vi "test Shutter.vi"() -> ()   [LabVIEW 2014]
doc: "Newport Motion Controler\nThis program test Shutter operations\n\nAndré Romero - 2020\nandretec@ifsc.usp.br"
panel:
  in  "Stop Button":bool
  in  "toggle Shutter":bool
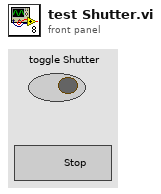
[diagram p1: front panel]
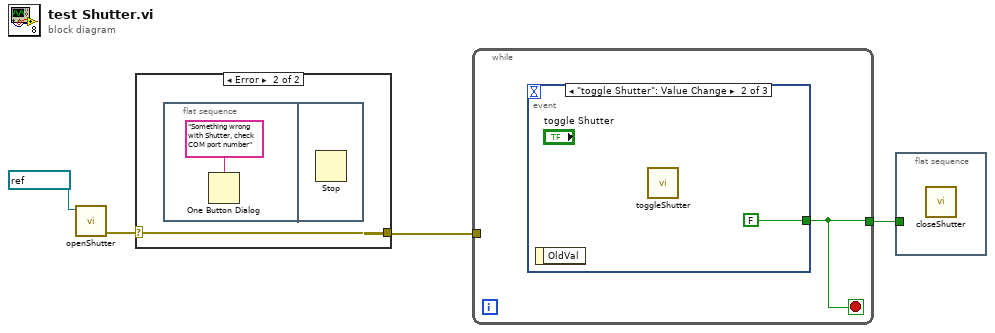
[diagram p0: block diagram]
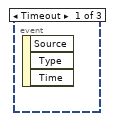
[diagram p2: hidden frame]
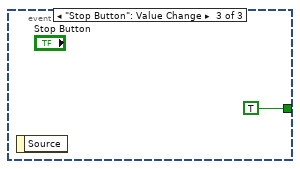
[diagram p3: hidden frame]
diagram:
  n1 = call "openShutter.vi"("VISA Refnum in"=refnum<visa-resource-name> "COM3") -> ("error out"=w3:errorcluster)  [unwired: 9 in, 1 out]
  n2 = case shown="Error" w3 {
    selector: w3 -> [w5 w6]
    tunnel: [w5 w6] -> w2
    frame No Error {
    }
    frame Error {
      n3 = flat-sequence {
        frame #0 {
          n4 = One Button Dialog(message="Something wrong with Shutter, check COM port number") -> ()  [unwired: 1 in, 1 out]
        }
        frame #1 {
          n5 = Stop() -> ()  [unwired: 1 in]
        }
      }
    }
  }
  n6 = while {
    tunnel: w2 -> [_]
    tunnel: [w8] -> w1
    stop <- w8 stop-if-true
    n7 = event shown="[1] \"toggle Shutter\": Value Change" {
      selector: _ -> [_ _ _]
      dyn-events: _ -> [_ _ _]
      timeout: _ -> [_ _ _]
      tunnel: [_ FALSE TRUE] -> w8
      event Timeout {
        n8 = event-data() -> ()  [unwired: 1 in, 3 out]
      }
      event "toggle Shutter": Value Change {
        n9 = event-data() -> ()  [unwired: 1 in, 1 out]
        n10 = call "toggleShutter.vi"() -> ()  [unwired: 10 in, 1 out]
      }
      event "Stop Button": Value Change {
        n11 = event-data() -> ()  [unwired: 1 in, 1 out]
      }
    }
  }
  n12 = flat-sequence {
    tunnel: w1 -> [_]
    frame #0 {
      n13 = call "closeShutter.vi"() -> ()  [unwired: 11 in, 1 out]
    }
  }
